vi "Init Amp2.vi"(8 "error in (no error)":errorcluster, 11 "VI Refnum":refnum<vi>) -> (0 "error out":errorcluster, 3 "VI out":refnum<vi>)   [LabVIEW 2020, in "BELLAxtalNathan.lvclass"]
uses:
  BELLAxtalNathan.lvclass
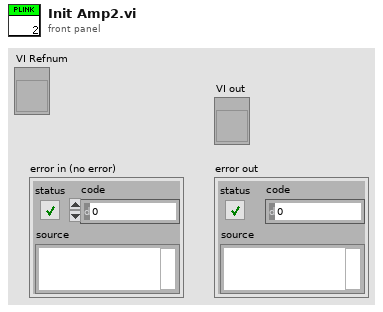
[diagram p1: front panel]
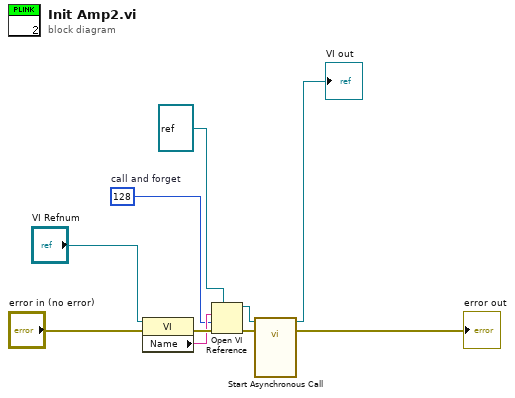
[diagram p0: block diagram]
diagram:
  w2 = 128  # call and forget
  n1 = property class="VI"(reference="VI Refnum", error in="error in (no error)") -> (error out=w6:errorcluster, "Name"=w5:string)  [unwired: 1 out]
  n2 = Open VI Reference(type specifier VI Refnum (for type only)=refnum<vi> refnum, vi path=w5, options=w2, error in (no error)=w6) -> (vi reference=w3:refnum<vi>, error out=w4:errorcluster)  [unwired: 2 in]
  n3 = call-by-ref "Start Asynchronous Call"(reference=w3, error in=w4) -> (reference out=→"VI out":refnum<vi>, error out=→"error out":errorcluster)  [unwired: 12 in]
